vi "Cleanup.vi"(8 "error in (no error)":errorcluster, 11 "2DArrayManager in":refnum<class "2DArrayManager.lvclass">) -> (0 "error out":errorcluster)   [LabVIEW 2020, in "OOPanel.lvlib" / "2DArrayManager.lvclass"]
uses:
  2DArrayManager.lvclass
  2DArrayManager.lvclass/2DArrayManager.ctl
  Manager/Manager.lvclass
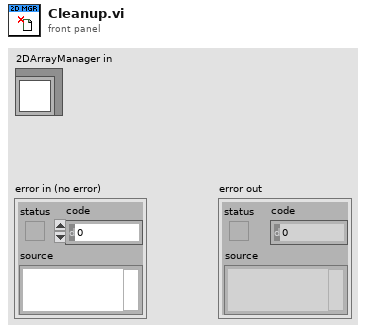
[diagram p1: front panel]
types:
  T1 = typedef "OOPanel.lvlib/2DArrayManager.lvclass/Events.ctl" = cluster{"Stop":refnum<user-event>, "Update":refnum<user-event>, "Set BG":refnum<user-event>, "Scroll":refnum<user-event>, "Highlight":refnum<user-event>, "Synced Scroll":refnum<user-event>}
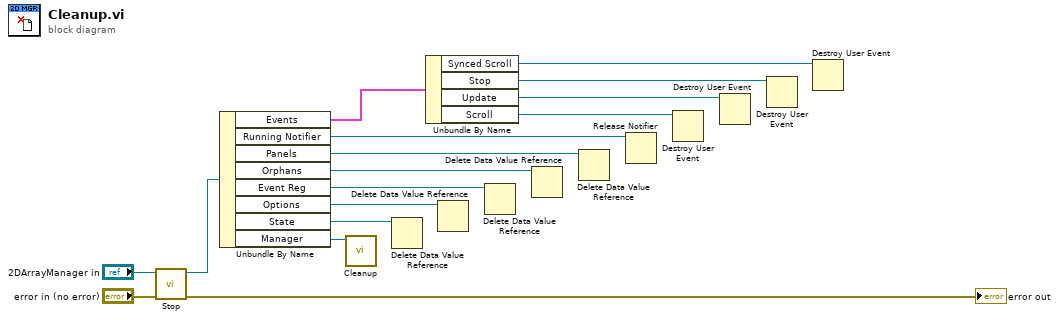
[diagram p0: block diagram]
diagram:
  n1 = call "Stop.vi"("error in (no error)"="error in (no error)", "2DArrayManager in"="2DArrayManager in") -> ("error out"=→"error out":errorcluster, "2DArrayManager out"=w13:refnum<class "2DArrayManager.lvclass">)  [unwired: 8 in]
  n2 = Unbundle By Name(w13) -> ("Events"=w6:T1, "Running Notifier"=w7:refnum<notifier>, "Panels"=w8:refnum<data-value>, "Orphans"=w9:refnum<data-value>, "Event Reg"=w10:refnum<data-value>, "Options"=w11:refnum<data-value>, "State"=w1:refnum<data-value>, "Manager"=w12:refnum<class "Manager.lvclass">)
  n3 = call "Cleanup.vi"("Manager in"=w12) -> ()  [unwired: 8 in, 3 out]
  n4 = Delete Data Value Reference(data value reference=w1) -> ()  [unwired: 1 in, 2 out]
  n5 = Unbundle By Name(w6) -> ("Synced Scroll"=w2:refnum<user-event>, "Stop"=w3:refnum<user-event>, "Update"=w4:refnum<user-event>, "Scroll"=w5:refnum<user-event>)
  n6 = Delete Data Value Reference(data value reference=w11) -> ()  [unwired: 1 in, 2 out]
  n7 = Delete Data Value Reference(data value reference=w10) -> ()  [unwired: 1 in, 2 out]
  n8 = Delete Data Value Reference(data value reference=w9) -> ()  [unwired: 1 in, 2 out]
  n9 = Delete Data Value Reference(data value reference=w8) -> ()  [unwired: 1 in, 2 out]
  n10 = Release Notifier(notifier=w7) -> ()  [unwired: 2 in, 3 out]
  n11 = Destroy User Event(user event=w5) -> ()  [unwired: 1 in, 1 out]
  n12 = Destroy User Event(user event=w4) -> ()  [unwired: 1 in, 1 out]
  n13 = Destroy User Event(user event=w3) -> ()  [unwired: 1 in, 1 out]
  n14 = Destroy User Event(user event=w2) -> ()  [unwired: 1 in, 1 out]
